vi "Assert Log File Is Valid.vi"(7 "Error":i32=10, 8 "error in":errorcluster, 9 "Expected Y Array Sizes":i32[](array[numeric])=[1000, 100], 10 "Expected Group dts":dbl[](array[numeric]), 11 "Embedded Data Logger System Tests in":refnum<class "Embedded Data Logger Windows System Tests.lvclass">) -> (0 "error out":errorcluster, 3 "Embedded Data Logger System Tests out":refnum<class "Embedded Data Logger Windows System Tests.lvclass">)   [LabVIEW 2027, in "Embedded Data Logger Windows System Tests.lvclass"]
uses:
  Embedded Data Logger Windows System Tests.lvclass
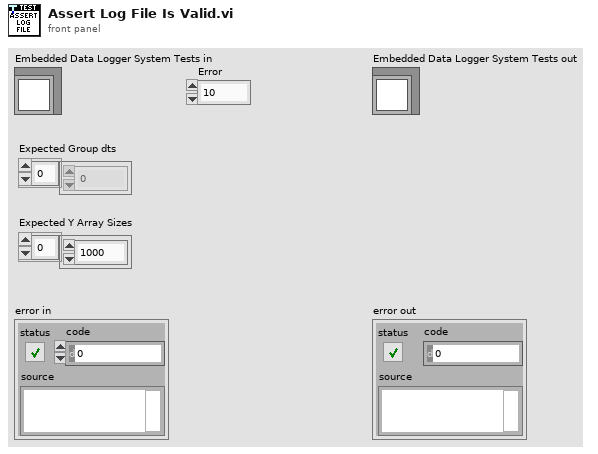
[diagram p1: front panel]
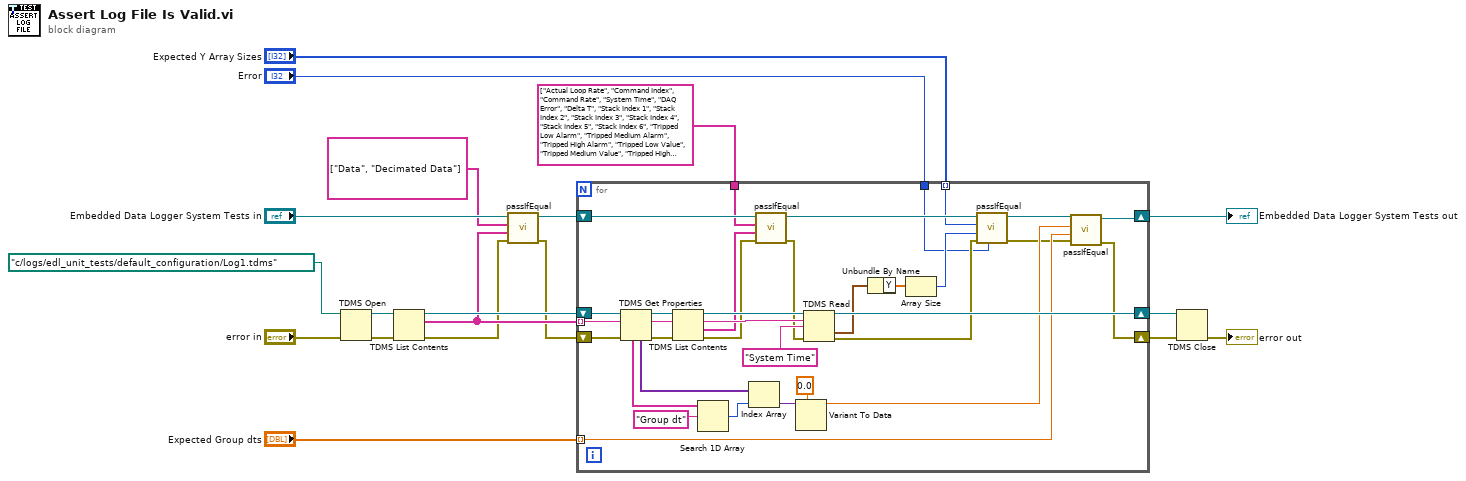
[diagram p0: block diagram]
diagram:
  n1 = TDMS Open(8:"error in", 11:path "c:/logs/edl_unit_tests/default_configuration/Log1.tdms" ("file path")) -> (0:w15:errorcluster, 3:w16:refnum<k34>)  [unwired: 5 in]
  n2 = TDMS List Contents(4:w15, 7:w16) -> (0:w5:errorcluster, 2:w6:string[], 3:w13:refnum<k34>)  [unwired: 1 in, 1 out]
  n3 = call-dynamic "passIfEqual.vi"("error in (no error)"=w5, "y"=w6, "x"=string[] ["Data", "Decimated Data"] ("group names"), "TestCase in"="Embedded Data Logger System Tests in") -> ("error out"=w4:errorcluster, "TestCase out"=w8:refnum<class "Embedded Data Logger Windows System Tests.lvclass">)  [unwired: 6 in]
  n4 = for {
    shift-right: [w24] -> w14
    shift-left: w4 -> [w23]
    shift-right: [w53] -> w12
    shift-left: w13 -> [w37]
    tunnel: w6 -> [w36] mode=indexing
    shift-right: [w26] -> w10
    shift-left: w8 -> [w51]
    tunnel: "Expected Y Array Sizes" -> [w40] mode=indexing
    tunnel: string[] ["Actual Loop Rate", "Command Index", "Command Rate", "System Time", "DAQ Error", "Delta T", "Stack Index 1", "Stack Index 2", "Stack Index 3", "Stack Index 4", "Stack Index 5", "Stack Index 6", "Tripped Low Alarm", "Tripped Medium Alarm", "Tripped High Alarm", "Tripped Low Value", "Tripped Medium Value", "Tripped High Value", "RT Engine Build", "HP Loop Duration", "LP Loop Duration", "System Command", "Streamed Channel Count", "Max Streamed Channels", "Model Count", "Maximum GENs", "Generator Engine State", "Watchdog Timer", "HS TCP Overflow Count", "Host IP", "Trace Enabled Flag", "Detailed Tracing Flag", "VI Tracing Flag", "Trace Buffer Size", "Thread Tracing Flag", "Absolute Time", "System Time - Microseconds", "ASAM XIL EESPort Trigger", "ASAM XIL EESPort Trigger Count", "Failure Count", "Analysis State", "TCP Data Packet Loss", "WPL Overflow Count", "WPL TCP Overflow Count", "WPL Error Count", "WPL Error Code", "Streamed Waveform Count", "Iteration", "Last Late Iteration", "Real-Time Sequence Command", "Real-Time Sequence Count", "HP Loop Wakeup Status", "HP-LP Overwrite", "LP Data Count", "HP Count", "LP Count", "Log Status"] ("channel names") -> [w44]
    tunnel: "Error" -> [w38]
    tunnel: "Expected Group dts" -> [w28] mode=indexing
    n5 = TDMS Get Properties(8:w23, 10:w36, 11:w37) -> (0:w20:errorcluster, 2:w22:string, 3:w21:refnum<k34>, 4:w33:variant[], 6:w35:string[])  [unwired: 3 in, 1 out]
    n6 = TDMS List Contents(4:w20, 6:w22, 7:w21) -> (0:w42:errorcluster, 1:w43:string[], 2:w46:string, 3:w47:refnum<k34>)
    n7 = Search 1D Array(1D array=w35, element="Group dt") -> (index of element=w32:i32)  [unwired: 1 in]
    n8 = Index Array(array=w33, index=w32) -> (element=w31:variant)
    n9 = call-dynamic "passIfEqual.vi"("error in (no error)"=w42, "y"=w43, "x"=w44, "TestCase in"=w51) -> ("error out"=w41:errorcluster, "TestCase out"=w45:refnum<class "Embedded Data Logger Windows System Tests.lvclass">)  [unwired: 6 in]
    n10 = Variant To Data(type=0.0, Variant=w31) -> (data=w29:dbl)  [unwired: 1 in, 1 out]
    n11 = TDMS Read(0:w47, 5:w46, 7:"System Time", 11:w41) -> (4:w53:refnum<k34>, 10:w50:waveform(dbl), 15:w48:errorcluster)  [unwired: 4 in, 3 out]
    n12 = Unbundle By Name(w50) -> ("Y"=w49:dbl[])
    n13 = Array Size(array=w49) -> (size(s)=w39:i32)
    n14 = call-dynamic "passIfEqual.vi"("delta (optional)"=w38, "error in (no error)"=w48, "y"=w39, "x"=w40, "TestCase in"=w45) -> ("error out"=w25:errorcluster, "TestCase out"=w27:refnum<class "Embedded Data Logger Windows System Tests.lvclass">)  [unwired: 5 in]
    n15 = call-dynamic "passIfEqual.vi"("error in (no error)"=w25, "y"=w28, "x"=w29, "TestCase in"=w27) -> ("error out"=w24:errorcluster, "TestCase out"=w26:refnum<class "Embedded Data Logger Windows System Tests.lvclass">)  [unwired: 6 in]
  }
  "Embedded Data Logger System Tests out" <- w10
  n16 = TDMS Close(8:w14, 11:w12) -> (0:→"error out":errorcluster)  [unwired: 1 out]
